vi "Replace_Array_Subset_1D_Element.vi"(9 "Element RAS":i8, 10 "Index RAS1D":i32, 11 "RAS1D":i8[](array[numeric])=[100, -1, -2, 9, 10]) -> (3 "New Array RAS1D":i8[](array[numeric]))   [LabVIEW 2018]
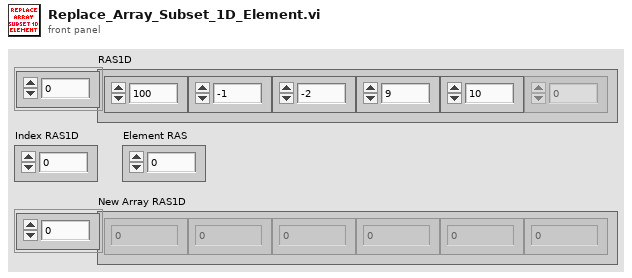
[diagram p1: front panel]
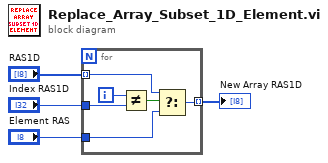
[diagram p0: block diagram]
diagram:
  n1 = for {
    tunnel: "RAS1D" -> [w10] mode=indexing
    tunnel: "Index RAS1D" -> [w7]
    tunnel: "Element RAS" -> [w6]
    tunnel: [w5] -> w4 mode=indexing
    i -> [w8]
    n2 = Not Equal?(x=w8, y=w7) -> (x != y?=w9:bool)
    n3 = Select(t=w10, s=w9, f=w6) -> (s? t:f=w5:i8)
  }
  "New Array RAS1D" <- w4
